vi "part2Rx.vi"() -> ()   [LabVIEW 2013]
uses:
  <instrlib>/niUSRP/niUSRP Fetch Rx Data (CDB Cluster).vi
panel:
  out "coerced gain":dbl format="%#_6f"
  out "coerced carrier frequency":dbl=100000.0 format="%#_6p"
  out "coerced IQ rate":dbl=100000.0 format="%#_6p"
  in  "active antenna":string
  in  "number of samples":i64=100000
  out "error out":errorcluster
  in  "gain":dbl format="%#_6f"
  in  "carrier frequency":dbl=100000.0 format="%#_6p"
  in  "IQ rate":dbl=100000.0 format="%#_6p"
  in  "USRP IP Address":refnum<k15>
  in  "stop":bool
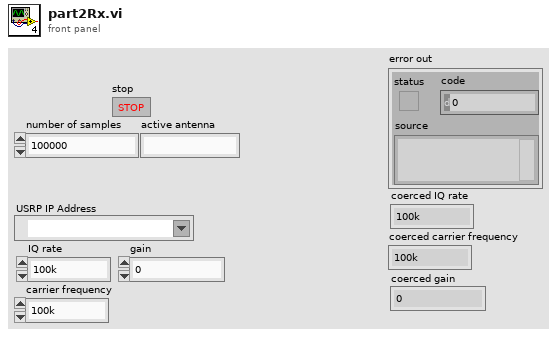
[diagram p1: front panel]
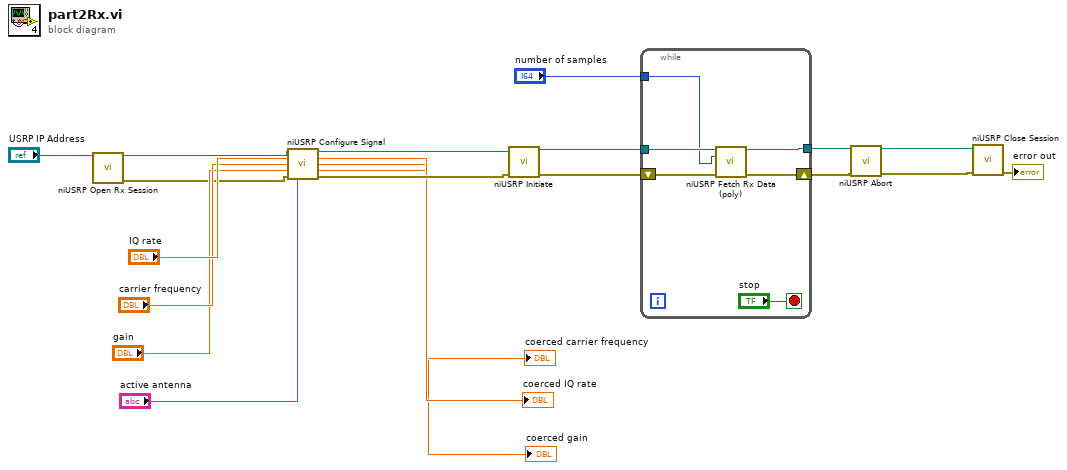
[diagram p0: block diagram]
diagram:
  n1 = call <instrlib>:"niUSRP Open Rx Session.vi"("device names"="USRP IP Address") -> ("session handle out"=w20:refnum<k15>, "error out"=w11:errorcluster)  [unwired: 13 in]
  n2 = call <instrlib>:"niUSRP Configure Signal.vi"("session handle"=w20, "IQ rate"="IQ rate", "carrier frequency"="carrier frequency", "gain"="gain", "error in (no error)"=w11, "active antenna"="active antenna") -> ("session handle out"=w19:refnum<k15>, "coerced IQ rate"=→"coerced IQ rate":dbl, "coerced carrier frequency"=→"coerced carrier frequency":dbl, "coerced gain"=→"coerced gain":dbl, "error out"=w10:errorcluster)  [unwired: 5 in]
  n3 = call <instrlib>:"niUSRP Initiate.vi"("session handle"=w19, "error in (no error)"=w10) -> ("session handle out"=w18:refnum<k15>, "error out"=w9:errorcluster)  [unwired: 12 in]
  n4 = while {
    tunnel: w18 -> [w26]
    tunnel: [w25] -> w17
    tunnel: "number of samples" -> [w21]
    shift-right: [w22] -> w8
    shift-left: w9 -> [w23]
    stop <- "stop" stop-if-true
    n5 = call-poly <instrlib>:"niUSRP Fetch Rx Data (poly).vi"("session handle"=w26, "number of samples"=w21, "error in (no error)"=w23) -> ("session handle out"=w25:refnum<k15>, "error out"=w22:errorcluster)  [unwired: 9 in, 2 out]
  }
  n6 = call <instrlib>:"niUSRP Abort.vi"("session handle"=w17, "error in (no error)"=w8) -> ("session handle out"=w16:refnum<k15>, "error out"=w7:errorcluster)  [unwired: 12 in]
  n7 = call <instrlib>:"niUSRP Close Session.vi"("session handle"=w16, "error in (no error)"=w7) -> ("error out"=→"error out":errorcluster)  [unwired: 13 in]
